vi "TUNA TAIL hindbrain ACT.vi"(0 "Speed Input":dbl(slide) scale=0.0005..0.0025 scale format="%#.1g", 5 "Heading Input":dbl(slide) scale=0.0005..0.0025 scale format="%_1f", 7 "TAIL PERIOD":dbl=500.0, 9 "LOOPCOUNT IN":dbl min=-45.0 max=45.0 step=1.0, 11 "error in":errorcluster) -> (1 "Desired \nRudder":dbl, 3 "Rudder":dbl min=-45.0 max=45.0 step=1.0, 4 "Desired\nSpeed":dbl, 6 "error out":errorcluster, 10 "Desired Tail Position":dbl min=-9.0 max=9.0 step=1.0)   [LabVIEW 2014]
doc: "This vi has two functions: it selects between manual and auto mode and it converts the incoming value into speed and rudder control values."
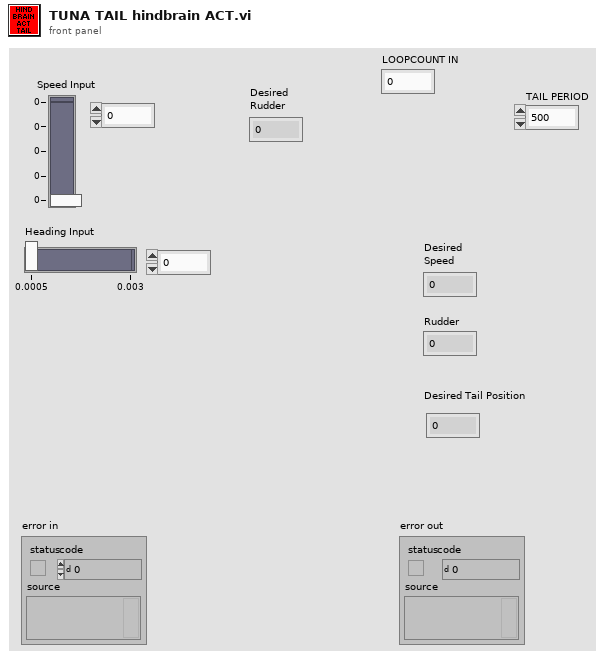
[diagram p1: front panel]
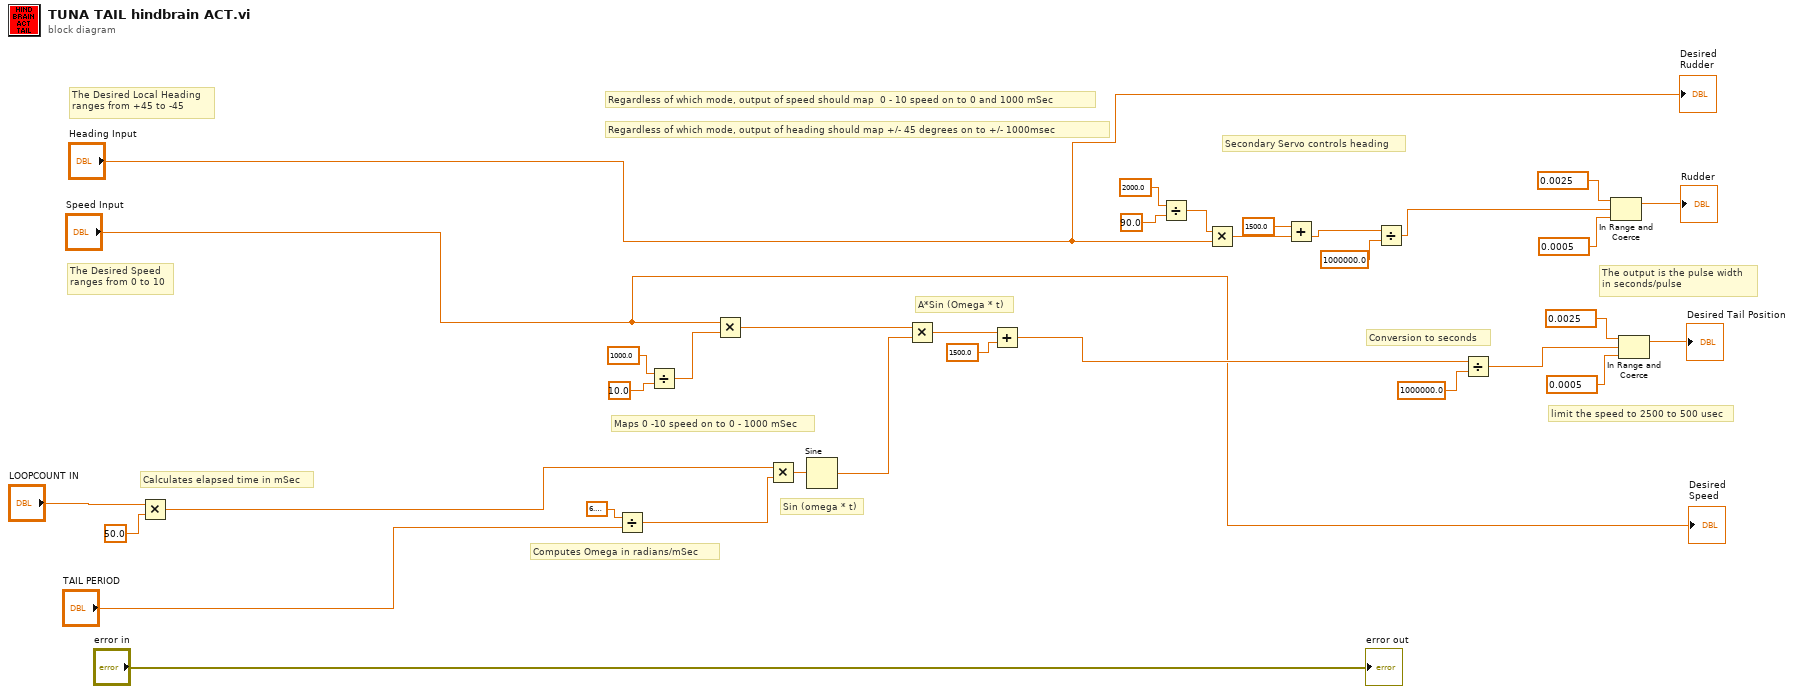
[diagram p0: block diagram]
diagram:
  # "A*Sin (Omega * t)"
  # "Sin (omega * t)"
  # "Maps 0 -10 speed on to 0 - 1000 mSec"
  # "Calculates elapsed time in mSec"
  # "Computes Omega in radians/mSec"
  # "Regardless of which mode, output of heading should map +/- 45 degrees on to +/- 1000msec"
  # "Regardless of which mode, output of speed should map  0 - 10 speed on to 0 and 1000 mSec"
  # "The Desired Local Heading\nranges from +45 to -45"
  # "The Desired Speed\nranges from 0 to 10"
  # "Conversion to seconds"
  # "Secondary Servo controls heading"
  # "The output is the pulse width\nin seconds/pulse"
  # "limit the speed to 2500 to 500 usec"
  n1 = Multiply(x="LOOPCOUNT IN", y=50.0) -> (x*y=w9:dbl)
  n2 = Divide(x=6.283185307179586, y="TAIL PERIOD") -> (x/y=w10:dbl)
  n3 = Divide(x=1000.0, y=10.0) -> (x/y=w12:dbl)
  n4 = Multiply(x="Speed Input", y=w12) -> (x*y=w7:dbl)
  n5 = Multiply(x=w9, y=w10) -> (x*y=w11:dbl)
  n6 = Sine(x=w11) -> (sin(x)=w8:dbl)
  n7 = Multiply(x=w7, y=w8) -> (x*y=w5:dbl)
  n8 = Add(x=w5, y=1500.0) -> (x+y=w4:dbl)
  n9 = Divide(x=2000.0, y=90.0) -> (x/y=w26:dbl)
  n10 = Multiply(x=w26, y="Heading Input") -> (x*y=w25:dbl)
  n11 = Add(x=1500.0, y=w25) -> (x+y=w20:dbl)
  n12 = Divide(x=w20, y=1000000.0) -> (x/y=w23:dbl)
  n13 = Divide(x=w4, y=1000000.0) -> (x/y=w21:dbl)
  n14 = In Range and Coerce(upper limit=0.0025 ("t"), x=w23, lower limit=0.0005 ("t")) -> (coerced(x)=→"Rudder":dbl)  [unwired: 1 out]
  n15 = In Range and Coerce(upper limit=0.0025 ("t"), x=w21, lower limit=0.0005 ("t")) -> (coerced(x)=→"Desired Tail Position":dbl)  [unwired: 1 out]
  "error out" <- "error in"
  "Desired \nRudder" <- "Heading Input"
  "Desired\nSpeed" <- "Speed Input"
